vi "Flatten Value.vi"(8 "Error In":errorcluster, 11 "Flt Array In":refnum<class "1D Flt.lvclass">) -> (0 "Error Out":errorcluster, 1 "Value":string, 3 "Flt Array Out":refnum<class "1D Flt.lvclass">)   [LabVIEW 2017, in "Tree API.lvlib" / "1D Flt.lvclass"]
uses:
  1D Flt.lvclass
  Tree Manager/Tree.lvclass
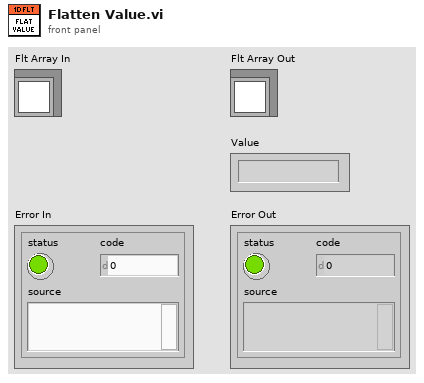
[diagram p1: front panel]
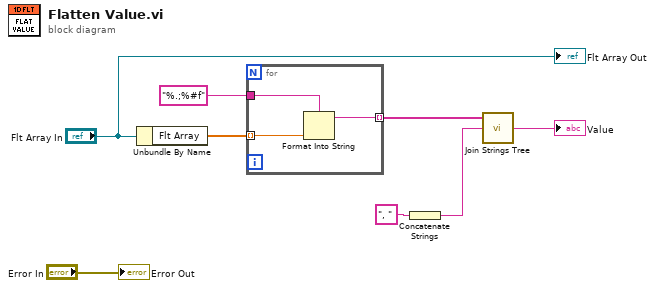
[diagram p0: block diagram]
diagram:
  n1 = Unbundle By Name("Flt Array In") -> ("Flt Array"=w7:dbl[])
  n2 = for {
    tunnel: w7 -> [w11] mode=indexing
    tunnel: [w10] -> w5 mode=indexing
    tunnel: "%.;%#f" ("initial string") -> [w9]
    n3 = Format Into String(format string=w9, w11) -> (resulting string=w10:string)  [unwired: 2 in, 1 out]
  }
  n4 = Concatenate Strings(", " ("Separator (,)")) -> (w2:string)
  n5 = call "Join Strings Tree.vi"("Separator (,)"=w2, "Strings In"=w5) -> ("String"=→"Value":string)  [unwired: 1 in]
  "Flt Array Out" <- "Flt Array In"
  "Error Out" <- "Error In"
